vi "Update Documentation Version.vi"(8 "error in (no error)":errorcluster, 9 "Description":string, 10 "Version":T1, 11 "LabVIEW Build Script in":refnum<class "LabVIEW Build Script.lvclass">) -> (0 "error out":errorcluster)   [LabVIEW 2021, in "LabVIEW Build Script.lvclass"]
uses:
  LabVIEW Build Script.lvclass
  <vilib>/CIF Foundation/CIF LabVIEW Scripting/LV Scripting/Typedef/Version.ctl
  LabVIEW Build Script.lvclass/LabVIEW Build Script.ctl
  Build Script Common/Typedef/Build Script Errors.ctl
  <vilib>/Utility/traverseref.llb/TRef TravTarget.ctl
  Accessors/Read VI Map.vi
  <vilib>/CIF Foundation/CIF Utilities/Errors/Append Error Location.vi
  Build Script Common/Build Script Common.lvlib
  <vilib>/Utility/traverseref.llb/VI Scripting - Traverse.lvlib
  <vilib>/CIF Foundation/CIF LabVIEW Scripting/LV Scripting/LV Scripting Utilities.lvlib
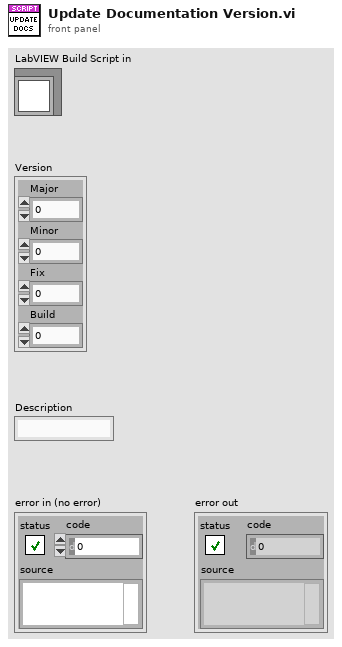
[diagram p1: front panel]
types:
  T1 = typedef "Version.ctl" = cluster{"Major":u16, "Minor":u16, "Fix":u16, "Build":u16}
  T2 = typedef "LV Scripting Utilities.lvlib/VI Map.ctl" = map{string, refnum<vi>}
  T3 = typedef "Build Script Common.lvlib/Build Script Errors.ctl" = enum16{"Item not found"}
  T4 = typedef "TRef TravTarget.ctl" = enum16{"FP", "BD", "Other"}
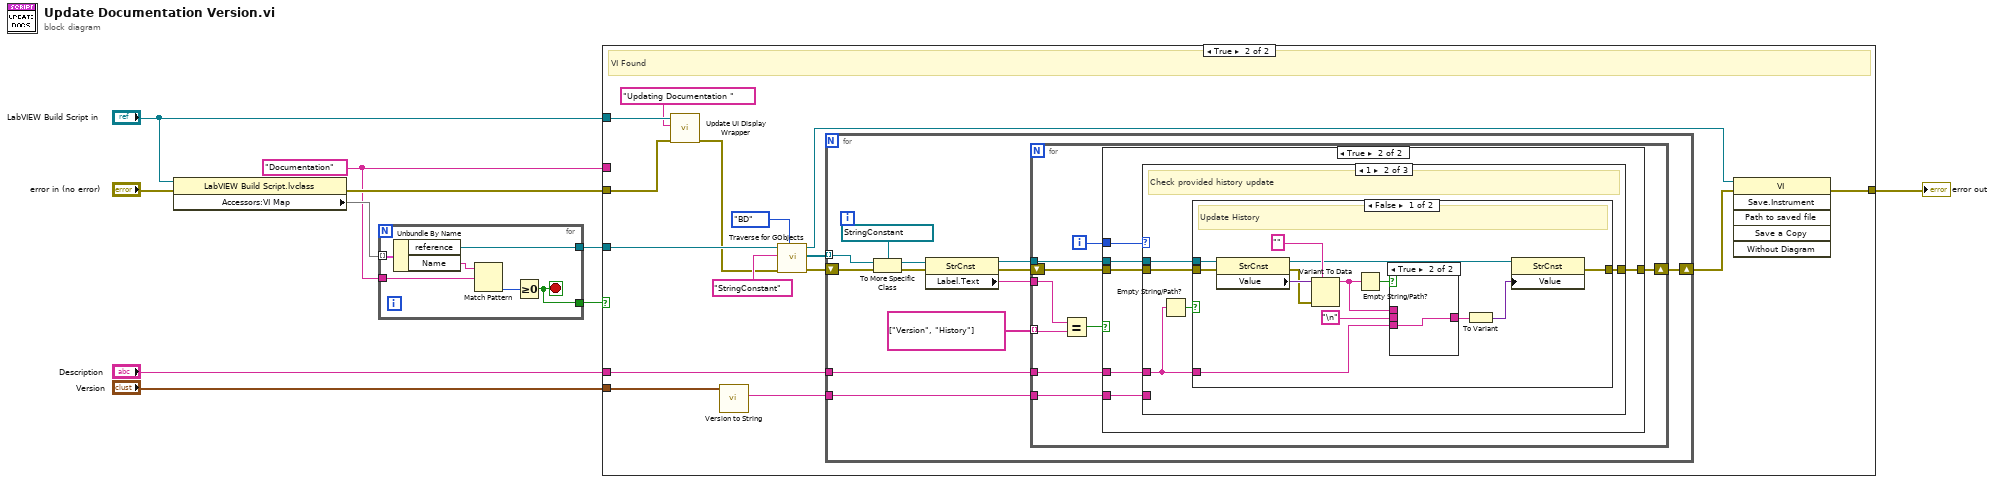
[diagram p0: block diagram]
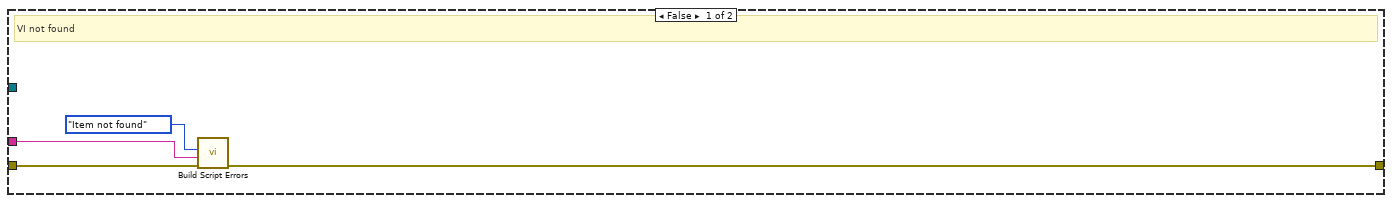
[diagram p2: hidden frame]
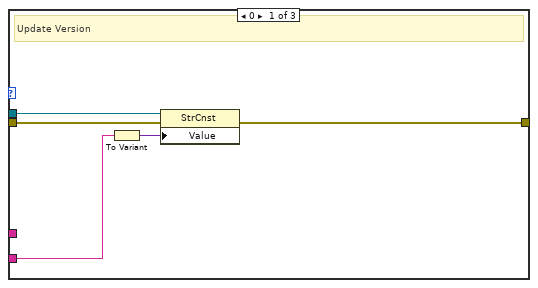
[diagram p4: hidden frame]
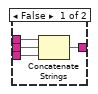
[diagram p5: hidden frame]
diagram:
  w2 = "Documentation" ("Search Pattern")
  n1 = property class="LabVIEW Build Script.lvclass"(reference="LabVIEW Build Script in", error in="error in (no error)") -> (error out=w8:errorcluster, "Accessors:VI Map"=w4:T2)  [unwired: 1 out]
  n2 = for {
    tunnel: w4 -> [w16] mode=indexing
    tunnel: w2 -> [w15]
    tunnel: [w12] -> w3
    tunnel: [w11] -> w1
    stop <- w12 stop-if-true
    n3 = Unbundle By Name(w16) -> ("reference"=w11:refnum<vi>, "Name"=w13:string)
    n4 = Match Pattern(string=w13, regular expression=w15) -> (offset past match=w14:i32)  [unwired: 1 in, 3 out]
    n5 = Greater Or Equal To 0?(x=w14) -> (x >= 0?=w12:bool)
  }
  n6 = case shown="True" w3 {
    tunnel: w8 -> [w20 w23]
    tunnel: w2 -> [w19 _]
    tunnel: [w18 w26] -> w5
    tunnel: "LabVIEW Build Script in" -> [_ w24]
    tunnel: "Version" -> [_ w32]
    tunnel: "Description" -> [_ w30]
    tunnel: w1 -> [_ w25]
    frame False {
      # "VI not found"
      n7 = call "Build Script Errors.vi"("error in (no error)"=w20, "String to Append"=w19, "Error"=Build_Script_Errors."Item not found") -> ("error out"=w18:errorcluster)  [unwired: 8 in]
    }
    frame True {
      # "VI Found"
      n8 = call "Update UI Display Wrapper.vi"("error in (no error)"=w23, "Update for Display"="Updating Documentation ", "LabVIEW Build Script in"=w24) -> ("error out"=w21:errorcluster)  [unwired: 8 in]
      n9 = call <vilib>:"Version to String.vi"("Version"=w32) -> ("Three Level Version String"=w31:string)  [unwired: 9 in, 1 out]
      n10 = call <vilib>:"Traverse for GObjects.vi"("Traverse Target"=TRef_TravTarget."BD", "error in (no error)"=w21, "Class Name"="StringConstant", "VI Refnum"=w25) -> ("error out"=w29:errorcluster, "References"=w33:refnum<vi>[], "dup VI Refnum"=w28:refnum<vi>)  [unwired: 4 in, 1 out]
      n11 = for {
        tunnel: w33 -> [w47] mode=indexing
        tunnel: w31 -> [w40]
        shift-right: [w42] -> w27
        shift-left: w29 -> [w38]
        tunnel: w30 -> [w36]
        n12 = To More Specific Class(target class=refnum<vi> refnum ("x"), reference=w47, error in=w38) -> (specific class reference=w41:refnum<vi>, error out=w45:errorcluster)
        n13 = property class="StrCnst"(reference=w41, error in=w45) -> (reference out=w43:refnum<vi>, error out=w44:errorcluster, "Label.Text"=w39:string)
        n14 = for {
          tunnel: w43 -> [w55]
          tunnel: w40 -> [w53]
          tunnel: w39 -> [w50]
          shift-right: [w54] -> w42
          shift-left: w44 -> [w56]
          tunnel: string[] ["Version", "History"] -> [w52] mode=indexing
          tunnel: w36 -> [w48]
          i -> [w49]
          n15 = Equal?(x=w50, y=w52) -> (x = y?=w51:bool)
          n16 = case shown="True" w51 {
            tunnel: w56 -> [w57 w61]
            tunnel: w55 -> [_ w63]
            tunnel: [w57 w62] -> w54
            tunnel: w53 -> [_ w58]
            tunnel: w49 -> [_ w60]
            tunnel: w48 -> [_ w59]
            frame False {
            }
            frame True {
              n17 = case shown="1" w60 {
                tunnel: w63 -> [w68 w73 _]
                tunnel: [w64 w72 w93] -> w62
                tunnel: w61 -> [w67 w71 w93]
                tunnel: w59 -> [_ w69 _]
                tunnel: w58 -> [w65 _ _]
                frame 0 {
                  # "Update Version"
                  n18 = To Variant(anything=w65) -> (Variant=w66:variant)
                  n19 = property class="StrCnst"(reference=w68, error in=w67, "Value"=w66) -> (error out=w64:errorcluster)  [unwired: 1 out]
                }
                frame 1 {
                  # "Check provided history update"
                  n20 = Empty String/Path?(string/path=w69) -> (empty?=w70:bool)
                  n21 = case shown="False" w70 {
                    tunnel: w73 -> [w86 _]
                    tunnel: [w76 w92] -> w72
                    tunnel: w71 -> [w85 w92]
                    tunnel: w69 -> [w81 _]
                    frame False {
                      # "Update History"
                      n22 = property class="StrCnst"(reference=w86, error in=w85) -> (reference out=w78:refnum<vi>, error out=w83:errorcluster, "Value"=w84:variant)
                      n23 = Variant To Data(error in=w83, type="", Variant=w84) -> (data=w75:string)  [unwired: 1 out]
                      n24 = Empty String/Path?(string/path=w75) -> (empty?=w74:bool)
                      n25 = case shown="True" w74 {
                        tunnel: w81 -> [w90 w91]
                        tunnel: "\n" -> [w89 _]
                        tunnel: [w88 w91] -> w79
                        tunnel: w75 -> [w87 _]
                        frame False {
                          n26 = Concatenate Strings(w87, w89, w90) -> (w88:string)
                        }
                        frame True {
                        }
                      }
                      n27 = To Variant(anything=w79) -> (Variant=w77:variant)
                      n28 = property class="StrCnst"(reference=w78, "Value"=w77) -> (error out=w76:errorcluster)  [unwired: 1 in, 1 out]
                    }
                    frame True {
                      # "No update provided"
                    }
                  }
                }
                frame 2, Default {
                }
              }
            }
          }
        }
      }
      n29 = invoke class="VI" method="Save.Instrument"(reference=w28, error in=w27) -> (error out=w26:errorcluster)  [unwired: 4 in, 5 out]
    }
  }
  "error out" <- w5
